vi "TimeTag_LSW_edits_June 15.vi"() -> ()   [LabVIEW 2015]
doc: "This sample project is built upon the standard state machine template and shows how you could create an application that acquires, analyzes, and presents data. It includes functionality for presenting configuration dialogs, preserving settings between executions, loading and saving data, as well as exporting graph images and text files.\n\nIt is most appropriate for data that is acquired instantly as it does not allow for screen updates mid acquisition nor does it allow for continuous streaming to disk."
uses:
  <vilib>/ptbypt/NI_PtbyPt.lvlib
panel:
  in  "File Name 3":string="C:\\FPGA\\test.txt"
  in  "averaging points":dbl
  in  "Runs":dbl=100.0
  in  "Pulse TTL 2":bool
  in  "Pulse TTL 1":bool
  in  "Toggle\nTTL 2":bool
  in  "Toggle\nTTL 1":bool
  out "Total Starts":dbl
  in  "Record data":bool
  out "Initial time":dbl
  out "Elapsed time (s)":dbl
  out "FPGA_Run Status":dbl
  out "USB_Open Status":dbl
  out "Channel 4 Total\nCounts":dbl
  out "Channel 3 Total\nCounts":dbl
  out "Channel 2 Total\nCounts":dbl
  out "Channel 1 Total\nCounts":dbl
  in  "File Name":string="C:\\FPGA\\test.txt"
  out "?":dbl format="%#_4g"
  out "?":dbl
  out "?":dbl format="%#_4g"
  out "?":dbl
  out "stats":i64[](array[numeric])
  in  "Stop":bool
  out "Channel 4 CPS":dbl(knob) scale=0.0..600.0
  out "Channel 3 CPS":dbl(knob) scale=0.0..600.0
  out "Channel 2 CPS":dbl(knob) scale=0.0..600.0
  out "Channel 1 CPS":dbl(knob) scale=0.0..600.0
  # "Starts"
  # "Channel 1"
  # "Channel 2"
  # "Channel 3"
  # "Channel 4"
  # "Coincidence Channels 1 & 2"
  # "Coincidence Channels 1 & 3"
  # "Coincidence Channels 1 & 4"
  # "Coincidence Channels 2 & 3"
  # "Coincidence Channels 2 & 4"
  # "Coincidence Channels 3 & 4"
  # "Coincidence Channels 1 & 2 & 3"
  # "Coincidence Channels 1 & 2 & 4"
  # "Coincidence Channels 1 & 3 & 4"
  # "Coincidence Channels 2 & 3 & 4"
  # "Coincidence Channels 1 & 2 & 3 & 4"
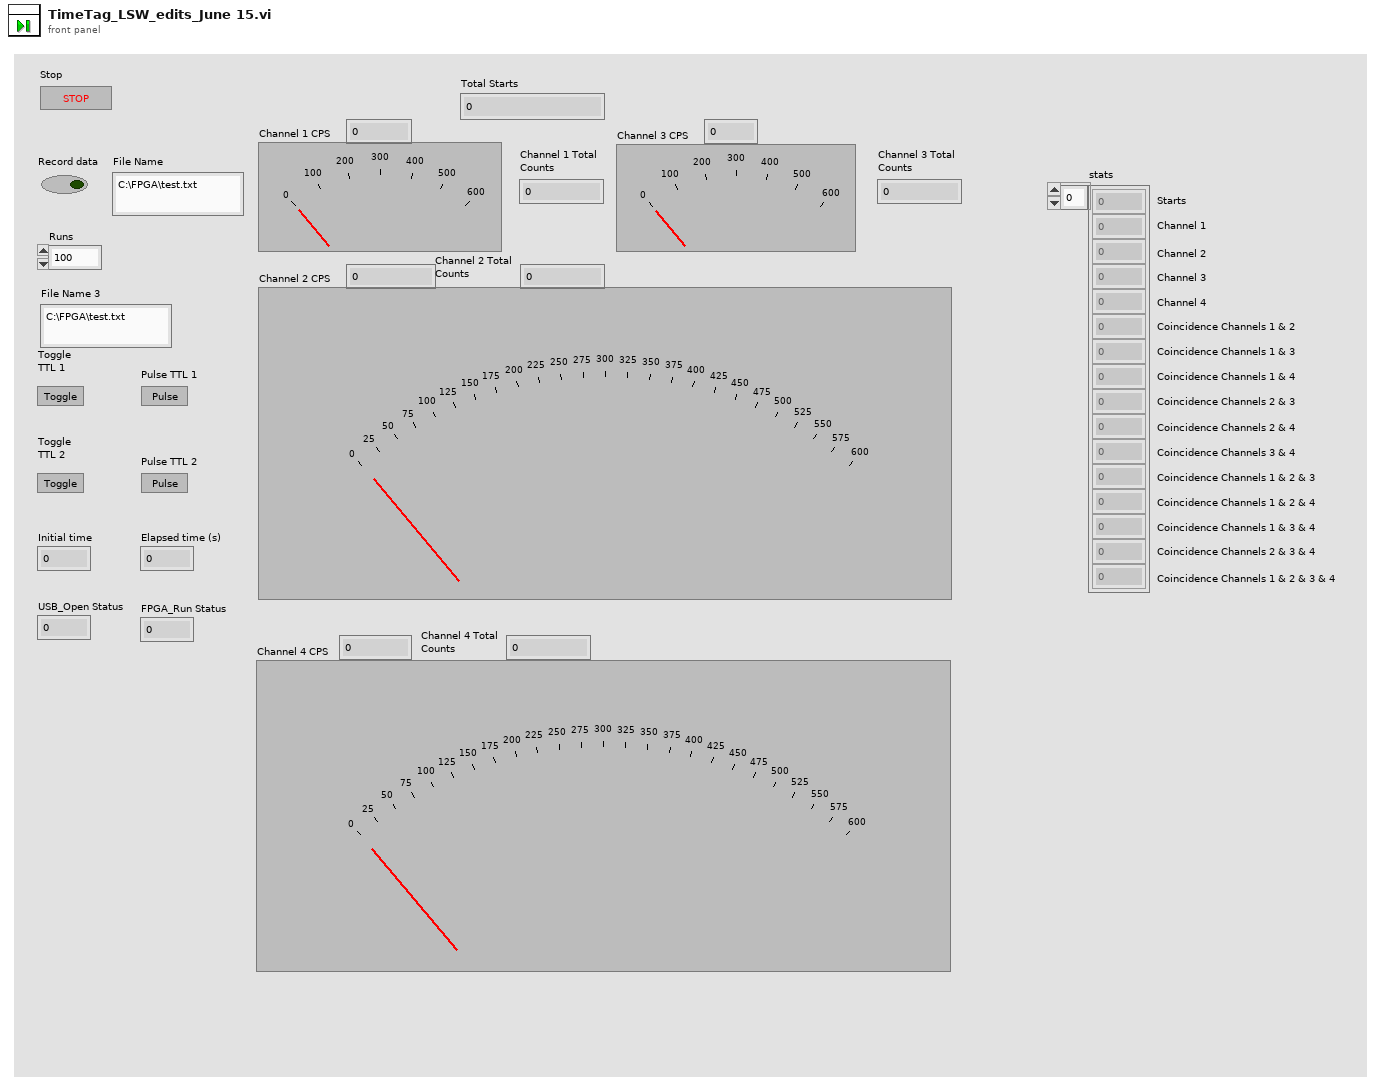
[diagram p1: front panel]
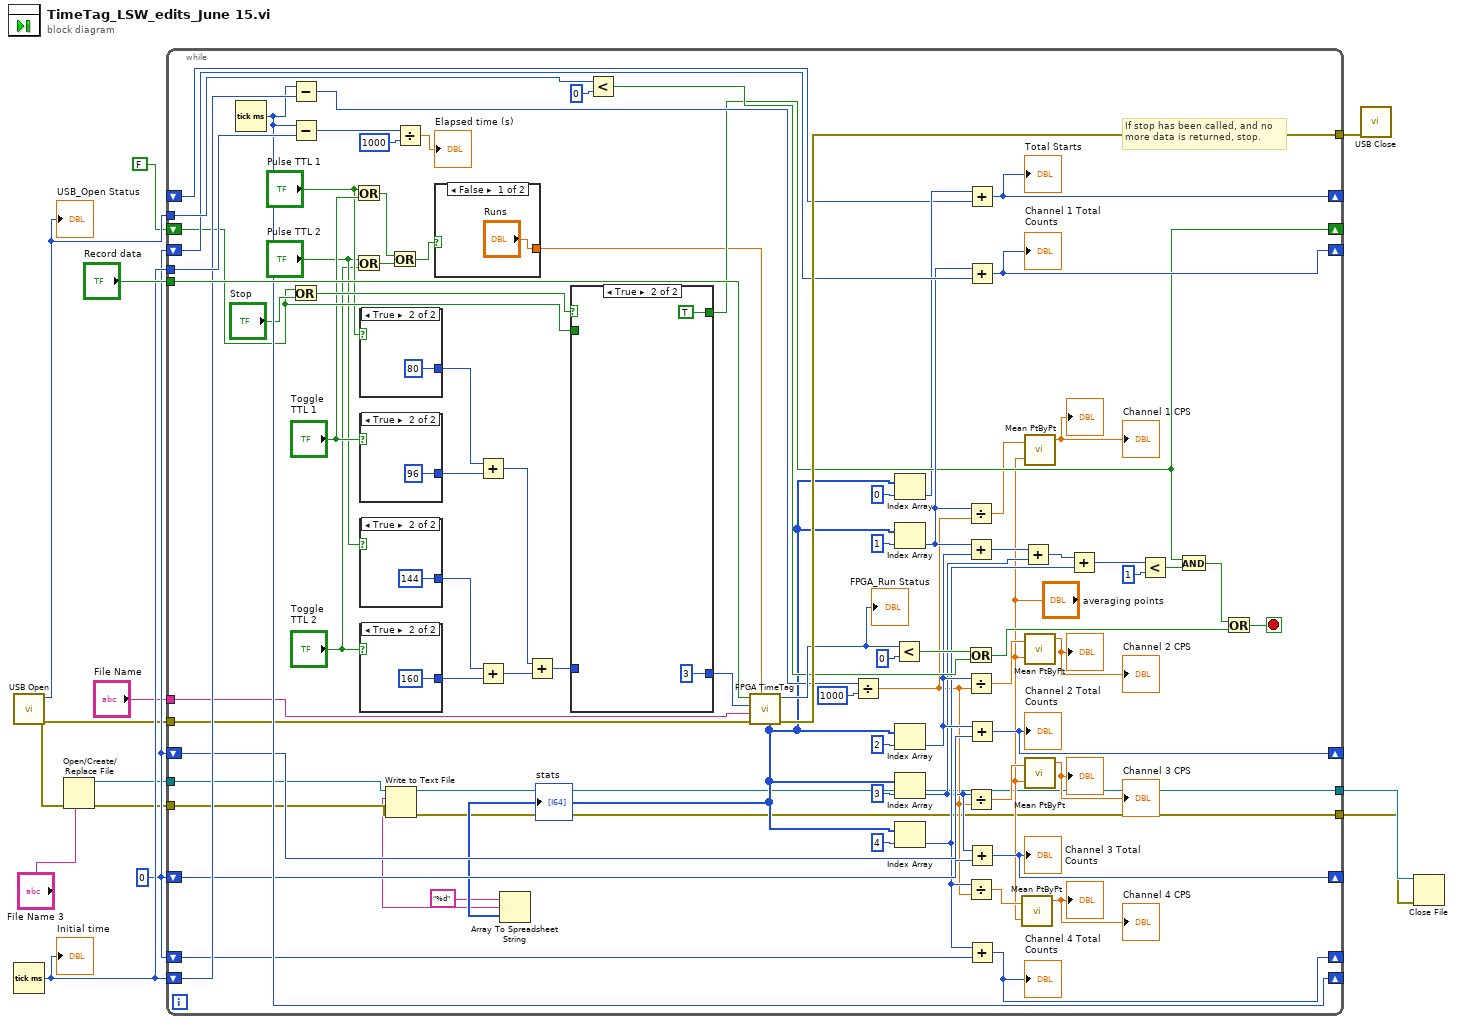
[diagram p0: block diagram]
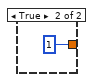
[diagram p2: hidden frame]
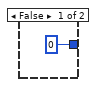
[diagram p3: hidden frame]
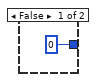
[diagram p4: hidden frame]
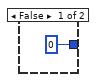
[diagram p5: hidden frame]
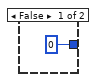
[diagram p6: hidden frame]
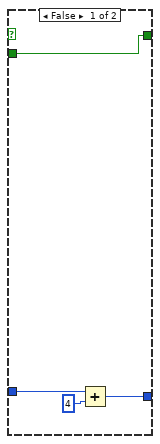
[diagram p7: hidden frame]
diagram:
  w9 = 0
  n1 = call "USB Open.vi"() -> ("error out"=w7:errorcluster, "function return"=w10:i32)  [unwired: 10 in]
  "USB_Open Status" <- w10
  n2 = Tick Count (ms)() -> (millisecond timer value=w11:u32)
  "Initial time" <- w11
  n3 = Open/Create/Replace File(error in=w7, prompt="File Name 3") -> (refnum out=w4:refnum<file>, error out=w3:errorcluster)  [unwired: 4 in, 1 out]
  n4 = while {
    tunnel: w11 -> [w96]
    shift-right: [w75] -> _
    shift-left: w9 -> [w70]
    shift-right: [w74] -> _
    shift-left: w9 -> [w69]
    shift-right: [w73] -> _
    shift-left: w9 -> [w68]
    shift-right: [w66] -> _
    shift-left: w9 -> [w67]
    tunnel: w7 -> [w21]
    tunnel: [w87] -> w12
    tunnel: "Record data" -> [w86]
    tunnel: "File Name" -> [w22]
    shift-right: [w71] -> _
    shift-left: w11 -> [w83]
    tunnel: w10 -> [w79]
    shift-right: [w55] -> _
    shift-left: FALSE -> [w52]
    shift-right: [w47] -> _
    shift-left: _ -> [w49]
    tunnel: w4 -> [w20]
    tunnel: w3 -> [w19]
    tunnel: [w15] -> w2
    tunnel: [w14] -> w1
    stop <- w88 stop-if-true
    # "If stop has been called, and no\nmore data is returned, stop."
    n5 = Tick Count (ms)() -> (millisecond timer value=w71:u32)
    n6 = Subtract(x=w71, y=w83) -> (x-y=w82:u32)
    n7 = Subtract(x=w71, y=w96) -> (x-y=w95:u32)
    n8 = Or(x=w52, y="Stop") -> (x .or. y?=w54:bool)
    n9 = Or(x="Pulse TTL 1", y="Toggle\nTTL 1") -> (x .or. y?=w38:bool)
    n10 = Or(x="Pulse TTL 2", y="Toggle\nTTL 2") -> (x .or. y?=w39:bool)
    n11 = case shown="True" "Pulse TTL 1" {
      tunnel: [0 80] -> w46
      frame False {
      }
      frame True {
      }
    }
    n12 = case shown="True" "Toggle\nTTL 1" {
      tunnel: [0 96] -> w45
      frame False {
      }
      frame True {
      }
    }
    n13 = case shown="True" "Pulse TTL 2" {
      tunnel: [0 144] -> w42
      frame False {
      }
      frame True {
      }
    }
    n14 = case shown="True" "Toggle\nTTL 2" {
      tunnel: [0 160] -> w43
      frame False {
      }
      frame True {
      }
    }
    n15 = Or(x=w38, y=w39) -> (x .or. y?=w40:bool)
    n16 = Divide(x=w95, y=1000) -> (x/y=→"Elapsed time (s)":dbl)
    n17 = case shown="False" w40 {
      tunnel: ["Runs" 1] -> w36
      frame False {
      }
      frame True {
      }
    }
    n18 = Add(x=w46, y=w45) -> (x+y=w44:i32)
    n19 = Add(x=w42, y=w43) -> (x+y=w41:i32)
    n20 = Add(x=w44, y=w41) -> (x+y=w37:i32)
    n21 = case shown="True" w54 {
      tunnel: [w108 3] -> w72
      tunnel: [w110 TRUE] -> w55
      tunnel: w52 -> [w110 _]
      tunnel: w37 -> [w107 _]
      frame False {
        n22 = Add(x=w107, y=4) -> (x+y=w108:i32)
      }
      frame True {
      }
    }
    n23 = Less?(x=w79, y=0) -> (x < y?=w77:bool)
    n24 = call "FPGA TimeTag.vi"("runs"=w36, "error in (no error)"=w21, "fileName"=w22, "fpgaCommand"=w72, "saveData"=w86) -> ("error out"=w87:errorcluster, "function return"=w85:i32, "stats"=w18:i64[])  [unwired: 4 in]
    "stats" <- w18
    "FPGA_Run Status" <- w85
    n25 = Array To Spreadsheet String(array=w18, 3:"%d") -> (spreadsheet string=w16:string)  [unwired: 1 in]
    n26 = Write to Text File(file (use dialog)=w20, text=w16, error in=w19) -> (refnum out=w15:refnum<file>, error out=w14:errorcluster)  [unwired: 1 in, 1 out]
    n27 = Divide(x=w82, y=1000) -> (x/y=w48:dbl)
    n28 = Less?(x=w85, y=0) -> (x < y?=w78:bool)
    n29 = Index Array(array=w18, index=0) -> (element=w50:i64)
    n30 = Index Array(array=w18, index=1) -> (element=w58:i64)
    n31 = Index Array(array=w18, index=2) -> (element=w65:i64)
    n32 = Index Array(array=w18, index=3) -> (element=w61:i64)
    n33 = Index Array(array=w18, index=4) -> (element=w62:i64)
    n34 = Divide(x=w58, y=w48) -> (x/y=w31:dbl)
    n35 = Add(x=w58, y=w65) -> (x+y=w60:i64)
    n36 = Or(x=w78, y=w77) -> (x .or. y?=w76:bool)
    n37 = Divide(x=w65, y=w48) -> (x/y=w29:dbl)
    n38 = Divide(x=w61, y=w48) -> (x/y=w27:dbl)
    n39 = Divide(x=w62, y=w48) -> (x/y=w25:dbl)
    n40 = Add(x=w50, y=w49) -> (x+y=w47:i64)
    "Total Starts" <- w47
    n41 = Add(x=w58, y=w70) -> (x+y=w75:i64)
    "Channel 1 Total\nCounts" <- w75
    n42 = Add(x=w65, y=w69) -> (x+y=w74:i64)
    "Channel 2 Total\nCounts" <- w74
    n43 = Add(x=w61, y=w68) -> (x+y=w73:i64)
    "Channel 3 Total\nCounts" <- w73
    n44 = Add(x=w62, y=w67) -> (x+y=w66:i64)
    "Channel 4 Total\nCounts" <- w66
    n45 = call <vilib>:"Mean PtByPt.vi"("x"=w25, "sample length"="averaging points") -> ("mean"=→"Channel 4 CPS" →"?":dbl)  [unwired: 2 in, 1 out]
    n46 = Add(x=w60, y=w61) -> (x+y=w64:i64)
    n47 = call <vilib>:"Mean PtByPt.vi"("x"=w31, "sample length"="averaging points") -> ("mean"=→"Channel 1 CPS" →"?":dbl)  [unwired: 2 in, 1 out]
    n48 = call <vilib>:"Mean PtByPt.vi"("x"=w29, "sample length"="averaging points") -> ("mean"=→"Channel 2 CPS" →"?":dbl)  [unwired: 2 in, 1 out]
    n49 = call <vilib>:"Mean PtByPt.vi"("x"=w27, "sample length"="averaging points") -> ("mean"=→"Channel 3 CPS" →"?":dbl)  [unwired: 2 in, 1 out]
    n50 = Add(x=w64, y=w62) -> (x+y=w63:i64)
    n51 = Less?(x=w63, y=1) -> (x < y?=w57:bool)
    n52 = And(x=w55, y=w57) -> (x .and. y?=w56:bool)
    n53 = Or(x=w56, y=w76) -> (x .or. y?=w88:bool)
  }
  n54 = call "USB Close.vi"("error in (no error)"=w12) -> ()  [unwired: 9 in, 2 out]
  n55 = Close File(refnum=w2, error in=w1) -> ()  [unwired: 2 out]
